vi "保存.vi"(7 "文件夹路径":path caption="路径", 8 "error in (no error)":errorcluster caption="错误输入（无错误）", 9 "激励信号":waveform(dbl), 10 "采集信号":waveform(dbl) caption="响应信号", 11 "文件类型":u16(ring)=2 items=["txt", "xls", "csv", "xlsx"]) -> (0 "error out":errorcluster caption="错误输出")   [LabVIEW 2018]
uses:
  <vilib>/Utility/file.llb/Write Delimited Spreadsheet (string).vi
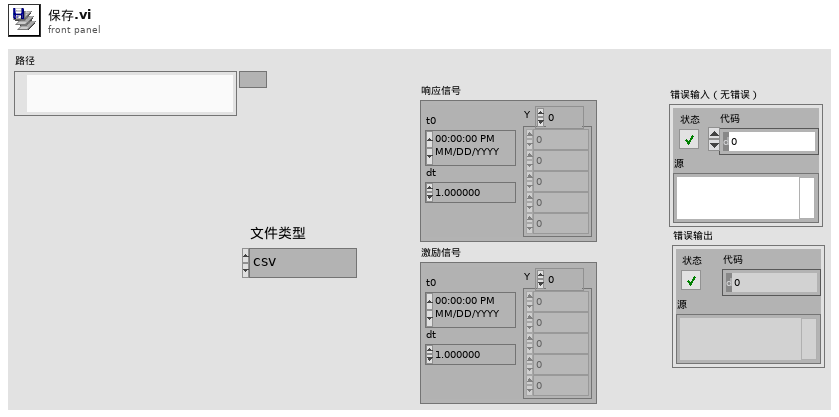
[diagram p1: front panel]
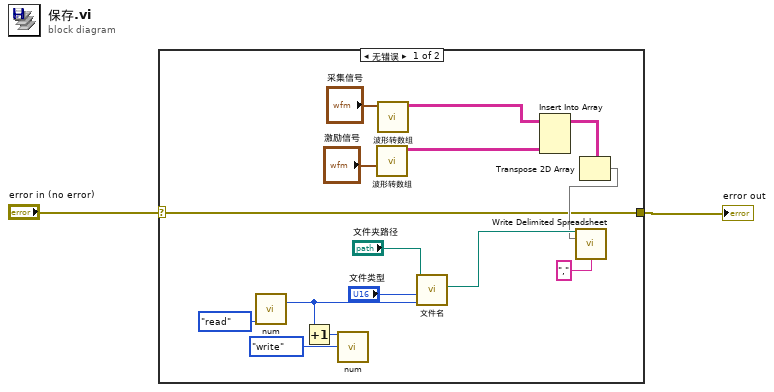
[diagram p0: block diagram]
diagram:
  n1 = case shown="无错误" "error in (no error)" {
    selector: "error in (no error)" -> [w7 w18]
    tunnel: [w7 w18] -> w1
    frame No Error {
      n2 = call "num.vi"("枚举"=enum16{"write", "read"}."read") -> ("num"=w15:i32)  [unwired: 10 in]
      n3 = Increment(x=w15) -> (x+1=w14:i32)
      n4 = call "num.vi"("枚举"=enum16{"write", "read"}."write", "num"=w14) -> ()  [unwired: 9 in, 1 out]
      n5 = call "波形转数组.vi"("响应信号"="激励信号") -> ("数组"=w10:string[][])  [unwired: 10 in]
      n6 = call "波形转数组.vi"("响应信号"="采集信号") -> ("数组"=w5:string[][])  [unwired: 10 in]
      n7 = call "文件名.vi"("第n个文件"=w15, "文件类型"="文件类型", "文件夹路径"="文件夹路径") -> ("添加的路径"=w12:path)  [unwired: 8 in]
      n8 = Insert Into Array(array=w5, new element=w10) -> (w9:string[][])  [unwired: 2 in]
      n9 = Transpose 2D Array(2D array=w9) -> (transposed array=w8:string[][])
      n10 = call-poly <vilib>:"Write Delimited Spreadsheet.vi"("file path (dialog if empty)"=w12, "2D data"=w8, "delimiter (\\t)"="," ("delimiter (\\t)")) -> ()  [unwired: 11 in, 2 out]
    }
    frame Error {
    }
  }
  "error out" <- w1
